vi "Append Digital Data By Sample.vi"() -> ()   [LabVIEW 2023]
doc: "This example illustrates how to append separate digital samples into one Digital Waveform.\n\nThe front panel has three digital controls that can be interactively edited by the user. The combined signals are displayed both numerically and graphically."
uses:
  <vilib>/Waveform/DTblOps.llb/DTbl Append Digital Samples.vi
panel:
  out "Digital Data Output":digitaldata
  in  "Digital Data 3":digitaldata={"transitions"=[], "data"=[[0, 0, 0, 0, 1, 1], [0, 0, 1, 0, 0, 1], [1, 0, 1, 0, 1, 0]]}
  in  "Digital Data 2":digitaldata={"transitions"=[], "data"=[[0, 0, 0, 0, 1, 0], [0, 0, 0, 1, 0, 1], [1, 0, 1, 0, 1, 0]]}
  in  "Digital Data 1":digitaldata={"transitions"=[], "data"=[[0, 0, 0, 0, 1], [0, 0, 1, 0, 0], [1, 0, 1, 0, 1]]}
  out "Digital Waveform Graph":digitaldata(graph)
  # "Overview: Illustrates how to append separate digital samples into a single value.\nInstructions:\nRun the VI."
  # "The values of Digital Data 1, Digital Data 2, and Digital Data 3 are appended by sample, then displayed in the Digital Data Output and Digital Waveform Graph indicators."
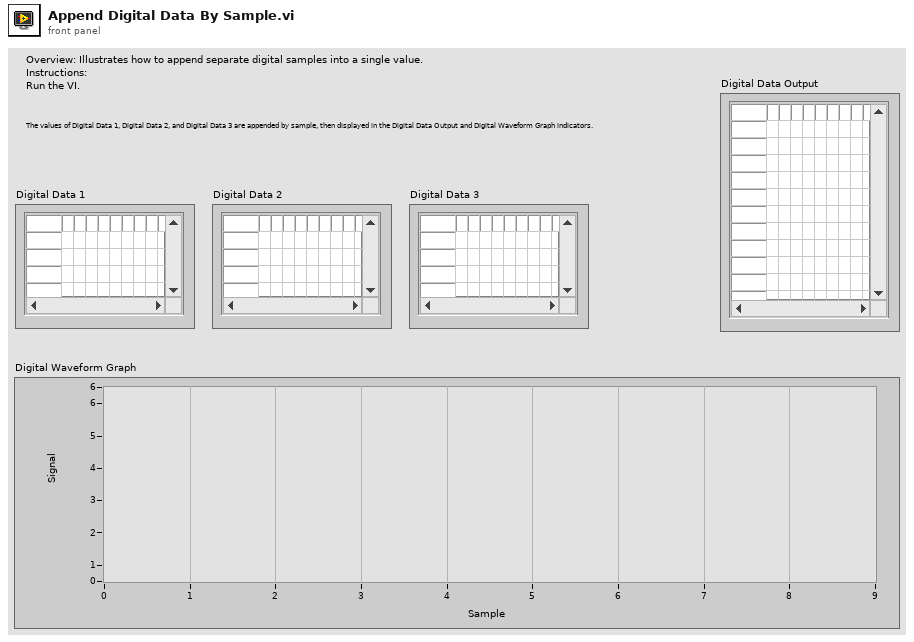
[diagram p1: front panel]
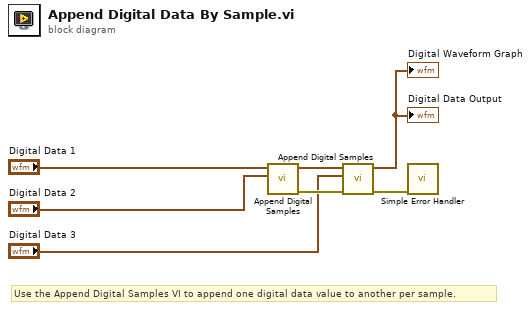
[diagram p0: block diagram]
diagram:
  # "Use the Append Digital Samples VI to append one digital data value to another per sample."
  n1 = call-poly <vilib>:"Append Digital Samples.vi"("digital data B"="Digital Data 2", "digital data A"="Digital Data 1") -> ("error out"=w7:errorcluster, "digital data out"=w2:digitaldata)  [unwired: 8 in]
  n2 = call-poly <vilib>:"Append Digital Samples.vi"("error in (no error)"=w7, "digital data B"="Digital Data 3", "digital data A"=w2) -> ("error out"=w6:errorcluster, "digital data out"=→"Digital Waveform Graph" →"Digital Data Output":digitaldata)  [unwired: 7 in]
  n3 = call <vilib>:"Simple Error Handler.vi"("error in (no error)"=w6) -> ()  [unwired: 4 in, 5 out]
